vi "notifyObservers.vi"(8 "error in (no error)":errorcluster, 11 "WeatherData in":refnum<class "Weather Station.lvclass">) -> (0 "error out":errorcluster, 3 "WeatherData out":refnum<class "Weather Station.lvclass">)   [LabVIEW 2020, in "Weather Station.lvclass"]
uses:
  Weather Station.lvclass
  Observable/Observable.lvclass
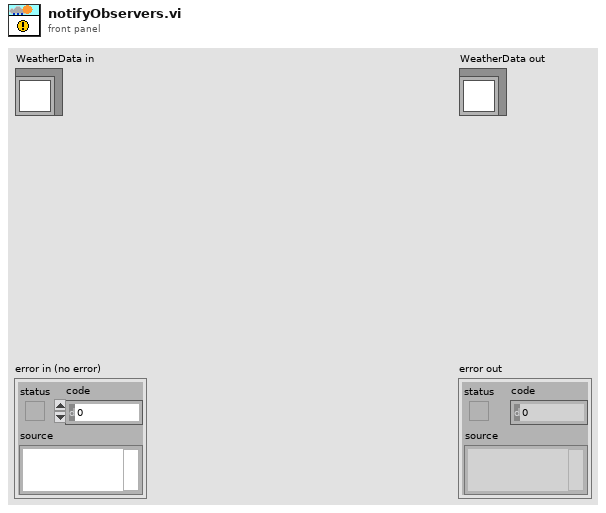
[diagram p1: front panel]
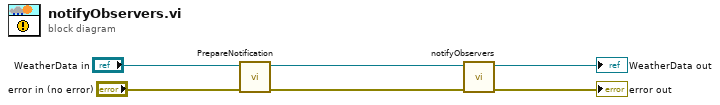
[diagram p0: block diagram]
diagram:
  n1 = call-dynamic "PrepareNotification.vi"("error in (no error)"="error in (no error)", "WeatherData in"="WeatherData in") -> ("error out"=w2:errorcluster, "WeatherData out"=w1:refnum<class "Weather Station.lvclass">)  [unwired: 8 in]
  n2 = call-parent "notifyObservers.vi"("error in (no error)"=w2, "Observable in"=w1) -> ("error out"=→"error out":errorcluster, "Observable out"=→"WeatherData out":refnum<class "Weather Station.lvclass">)  [unwired: 8 in]
